vi "loop error, restart vi.vi"(11 "error?":bool) -> ()   [LabVIEW 2013]
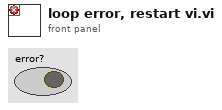
[diagram p1: front panel]
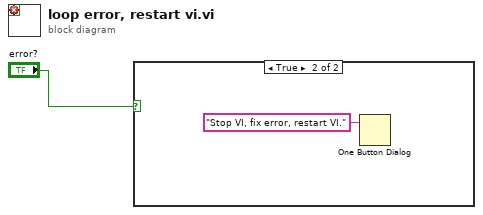
[diagram p0: block diagram]
diagram:
  n1 = case shown="True" "error?" {
    frame False {
    }
    frame True {
      n2 = One Button Dialog(message="Stop VI, fix error, restart VI.") -> ()  [unwired: 1 in, 1 out]
    }
  }
